vi "Workdays Count.vi"(10 "Since":timestamp format="%<%x>T", 11 "To":timestamp format="%<%x>T") -> (2 "work days":i32, 3 "Days":i32)   [LabVIEW 2018]
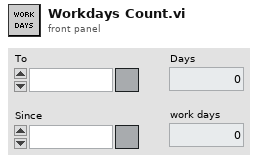
[diagram p1: front panel]
types:
  T1 = typedef "LVDateTimeRec.ctl" = cluster{"fractional second":dbl, "second":i32, "minute":i32, "hour":i32, "day of month":i32, "month":i32, "year":i32, "day of week":i32, "day of year":i32, "DST":i32}
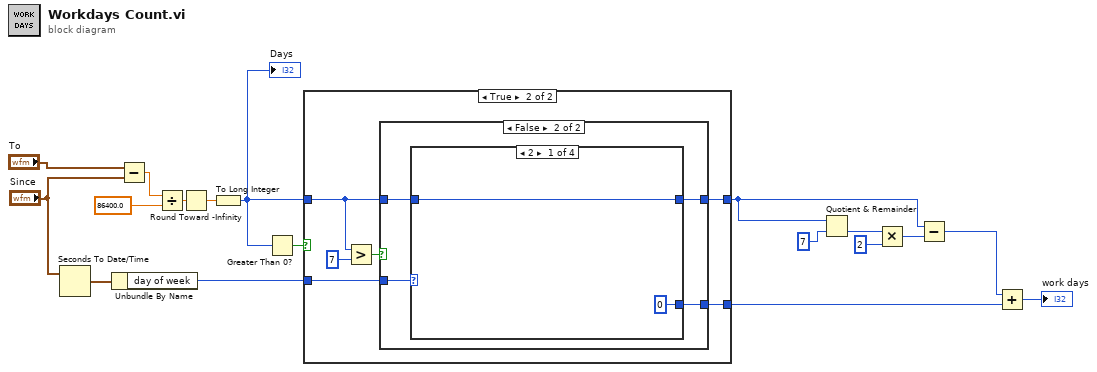
[diagram p0: block diagram]
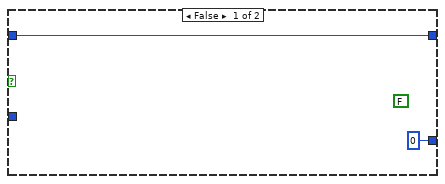
[diagram p2: hidden frame]
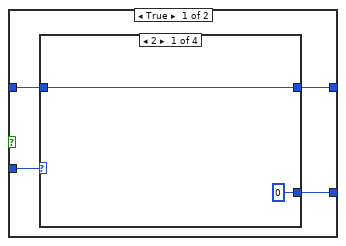
[diagram p3: hidden frame]
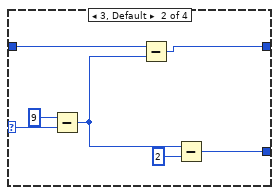
[diagram p4: hidden frame]
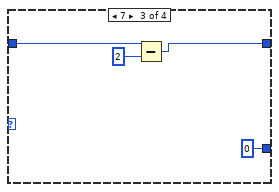
[diagram p5: hidden frame]
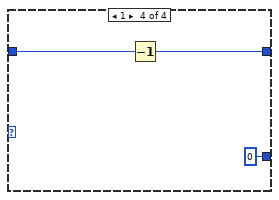
[diagram p6: hidden frame]
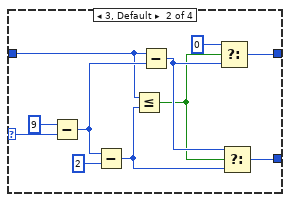
[diagram p7: hidden frame]
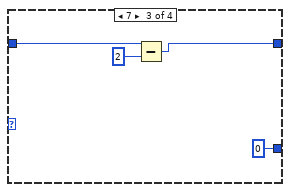
[diagram p8: hidden frame]
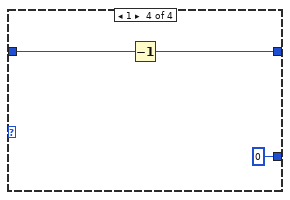
[diagram p9: hidden frame]
diagram:
  n1 = Seconds To Date/Time(time stamp (now)="Since") -> (date time rec=w8:T1)  [unwired: 1 in]
  n2 = Unbundle By Name(w8) -> ("day of week"=w9:i32)
  n3 = Subtract(x="To", y="Since") -> (x-y=w4:dbl)
  n4 = Divide(x=w4, y=86400.0) -> (x/y=w2:dbl)
  n5 = Round Toward -Infinity(1:w2) -> (0:w1:dbl)
  n6 = To Long Integer(number=w1) -> (32bit integer=w10:i32)
  "Days" <- w10
  n7 = Greater Than 0?(x=w10) -> (x > 0?=w5:bool)
  n8 = case shown="True" w5 {
    tunnel: w9 -> [_ w26]
    tunnel: w10 -> [w19 w24]
    tunnel: [w19 w25] -> w17
    tunnel: [0 w21] -> w16
    frame False {
      (unwired) FALSE ("s")
    }
    frame True {
      n9 = Greater?(x=w24, y=7) -> (0:w22:bool)
      n10 = case shown="False" w22 {
        tunnel: w26 -> [w30 w50]
        tunnel: [w29 w49] -> w25
        tunnel: w24 -> [w28 w48]
        tunnel: [w27 w47] -> w21
        frame True {
          n11 = case shown="2" w30 {
            selector: w30 -> [_ w36 _ _]
            tunnel: w28 -> [w32 w35 w42 w46]
            tunnel: [w32 w33 w41 w45] -> w29
            tunnel: [0 w37 0 0] -> w27
            frame 2 {
            }
            frame 3, Default {
              n12 = Subtract(x=9, y=w36) -> (x-y=w34:i32)
              n13 = Subtract(x=w35, y=w34) -> (x-y=w33:i32)
              n14 = Subtract(x=w34, y=2) -> (x-y=w37:i32)
            }
            frame 7 {
              n15 = Subtract(x=w42, y=2) -> (x-y=w41:i32)
            }
            frame 1 {
              n16 = Decrement(x=w46) -> (x-1=w45:i32)
            }
          }
        }
        frame False {
          n17 = case shown="2" w50 {
            selector: w50 -> [_ w61 _ _]
            tunnel: w48 -> [w52 w57 w66 w70]
            tunnel: [w52 w59 w65 w69] -> w49
            tunnel: [0 w58 0 0] -> w47
            frame 2 {
            }
            frame 3, Default {
              n18 = Subtract(x=9, y=w61) -> (x-y=w60:i32)
              n19 = Subtract(x=w60, y=2) -> (x-y=w56:i32)
              n20 = Less Or Equal?(x=w57, y=w56) -> (x <= y?=w53:bool)
              n21 = Subtract(x=w57, y=w60) -> (x-y=w55:i32)
              n22 = Select(t=0, s=w53, f=w55) -> (s? t:f=w59:i32)
              n23 = Select(t=w55, s=w53, f=w56) -> (s? t:f=w58:i32)
            }
            frame 7 {
              n24 = Subtract(x=w66, y=2) -> (x-y=w65:i32)
            }
            frame 1 {
              n25 = Decrement(x=w70) -> (x-1=w69:i32)
            }
          }
        }
      }
    }
  }
  n26 = Quotient & Remainder(x=w17, y=7) -> (floor(x/y)=w12:i32)  [unwired: 1 out]
  n27 = Multiply(x=w12, y=2) -> (x*y=w14:i32)
  n28 = Subtract(x=w17, y=w14) -> (x-y=w18:i32)
  n29 = Add(x=w18, y=w16) -> (x+y=→"work days":i32)
